vi "Board Type Enum To String.vi"(10 "Board Type":T1) -> (2 "String":string)   [LabVIEW 2011, in "LabVIEW Interface for ChipKit.lvlib"]
uses:
  LabVIEW Interface for ChipKit.lvlib
  Type Defs/Board Type.ctl
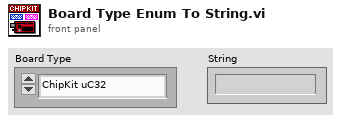
[diagram p1: front panel]
types:
  T1 = typedef "LabVIEW Interface for ChipKit.lvlib/Board Type.ctl" = enum16{"ChipKit uC32", "ChipKit Uno32", "ChipKit Max32"}
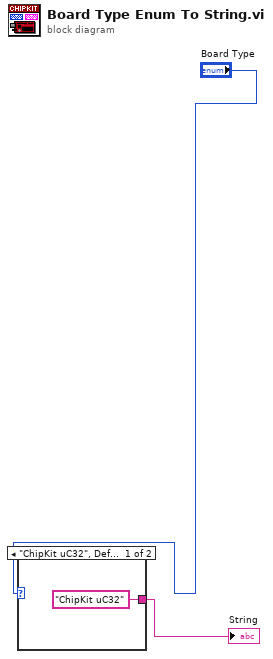
[diagram p0: block diagram]
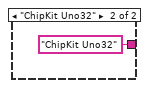
[diagram p2: hidden frame]
diagram:
  n1 = case shown="\"ChipKit uC32\", Default" "Board Type" {
    tunnel: ["ChipKit uC32" "ChipKit Uno32"] -> w2
    frame "ChipKit uC32", Default {
    }
    frame "ChipKit Uno32" {
    }
  }
  "String" <- w2
